vi "Log.vi"(7 "Source":string, 8 "error in (no error)":errorcluster, 9 "Message":string, 10 "Level":T1, 11 "Log Indicator In":refnum<class "Log Indicator.lvclass">) -> (0 "error out":errorcluster, 3 "Log Indicator Out":refnum<class "Log Indicator.lvclass">)   [LabVIEW 2020, in "Log Indicator.lvclass"]
doc: "Enter a message into the system log."
uses:
  Log Indicator.lvclass
  <vilib>/Astemes/Triarc Framework/Logging/Protected/Level.ctl
  Log Indicator.lvclass/Log Indicator.ctl
  <vilib>/Astemes/Triarc Framework/Logging/Logging.lvclass
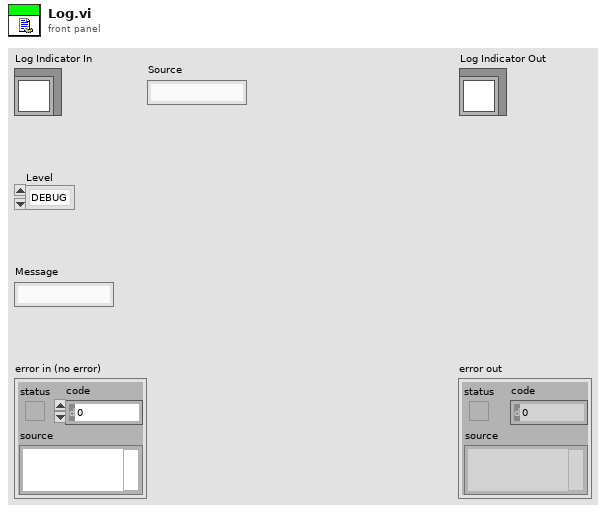
[diagram p1: front panel]
types:
  T1 = typedef "TF.lvlib/Logging.lvclass/Level.ctl" = enum16{"DEBUG", "INFO", "WARNING", "ERROR", "CRITICAL"}
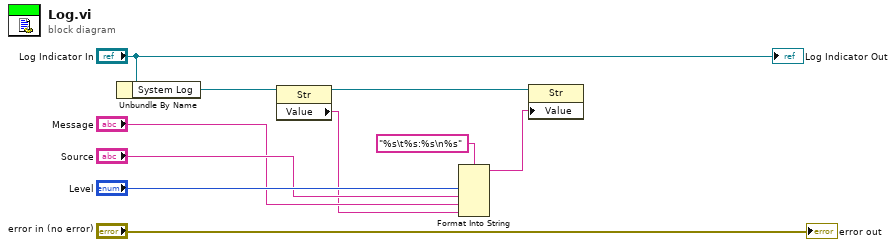
[diagram p0: block diagram]
diagram:
  n1 = Unbundle By Name("Log Indicator In") -> ("System Log"=w9:refnum<vi>)
  n2 = property class="Str"(reference=w9) -> (reference out=w8:refnum<vi>, "Value"=w3:string)  [unwired: 1 in, 1 out]
  n3 = Format Into String(format string="%s\t%s:%s\n%s", "Level", "Source", "Message", w3) -> (resulting string=w2:string)  [unwired: 2 in, 1 out]
  n4 = property class="Str"(reference=w8, "Value"=w2) -> ()  [unwired: 1 in, 2 out]
  "error out" <- "error in (no error)"
  "Log Indicator Out" <- "Log Indicator In"
